vi "SERIAL_CapturePacket.vi"(11 "Stream":string) -> (0 "Packet Located":bool, 1 "Packet Length":i32, 2 "Packet":string, 3 "Stream":string)   [LabVIEW 2014, in "navX-MXP IMU.lvlib"]
uses:
  navX-MXP IMU.lvlib
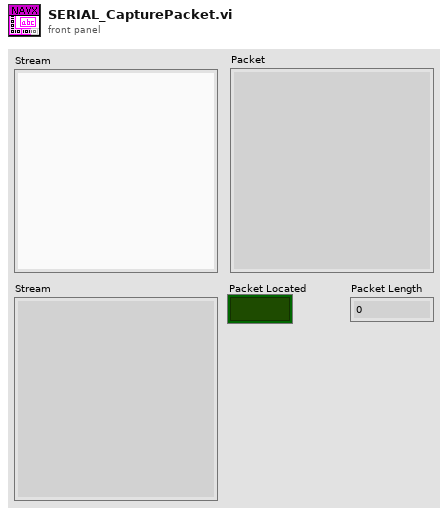
[diagram p1: front panel]
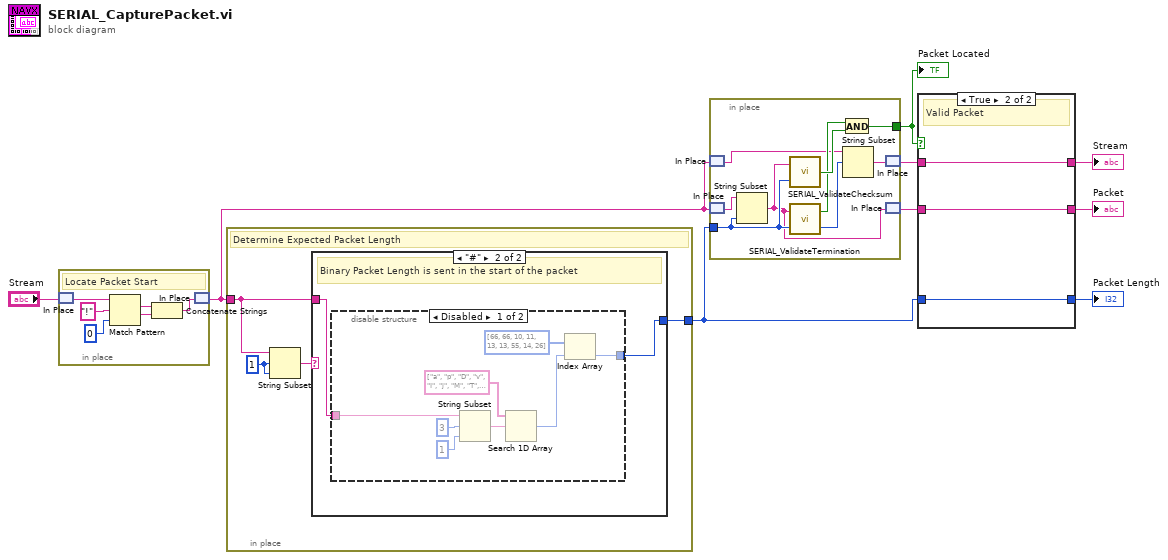
[diagram p0: block diagram]
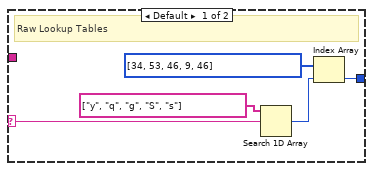
[diagram p2: hidden frame]
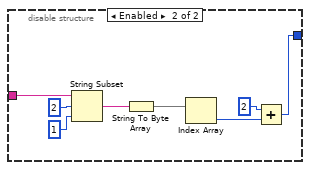
[diagram p3: hidden frame]
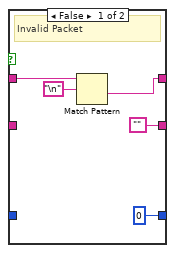
[diagram p4: hidden frame]
diagram:
  n1 = in-place {
    # "Locate Packet Start"
    n2 = in-place-match #1("Stream") -> (w11:string)
    n3 = Match Pattern(string=w11, regular expression="!" ("Packet Start Char"), offset (0)=0 ("offset past match")) -> (match substring=w14:string, after substring=w13:string)  [unwired: 2 out]
    n4 = Concatenate Strings(w14, w13) -> (w10:string)
    n5 = in-place-match #1(w10) -> (w3:string)
  }
  n6 = in-place {
    in-place-border: w3 -> [w18]
    in-place-border: [w17] -> w6
    w19 = 1 ("length (rest)")
    # "Determine Expected Packet Length"
    n7 = String Subset(string=w18, offset (0)=w19, length (rest)=w19) -> (substring=w16:string)
    n8 = case shown="\"#\"" w16 {
      selector: w16 -> [w20 _]
      tunnel: [w21 w26] -> w17
      tunnel: w18 -> [_ w25]
      frame Default {
        # "Raw Lookup Tables"
        n9 = Search 1D Array(1D array=string[] ["y", "q", "g", "S", "s"], element=w20) -> (index of element=w22:i32)  [unwired: 1 in]
        n10 = Index Array(array=i32[] [34, 53, 46, 9, 46], index=w22) -> (element=w21:i32)
      }
      frame "#" {
        # "Binary Packet Length is sent in the start of the packet"
        n11 = disable-structure shown="Disabled" {
          disable-tunnel: [w28 w35] -> w26
          disable-tunnel: w25 -> [w27 w36]
          frame Disabled {
            n12 = String Subset(string=w27, offset (0)=3, length (rest)=1 ("length (rest)")) -> (substring=w29:string)
            n13 = Search 1D Array(1D array=string[] ["a", "p", "D", "v", "I", "j", "M", "T", "i"], element=w29) -> (index of element=w34:i32)  [unwired: 1 in]
            n14 = Index Array(array=i32[] [66, 66, 10, 11, 13, 13, 55, 14, 26], index=w34) -> (element=w28:i32)
          }
          frame Enabled {
            n15 = String Subset(string=w36, offset (0)=2, length (rest)=1 ("length (rest)")) -> (substring=w39:string)
            n16 = String To Byte Array(string=w39) -> (unsigned byte array=w40:u8[])
            n17 = Index Array(array=w40) -> (element=w41:u8)  [unwired: 1 in]
            n18 = Add(x=u8 2 ("y"), y=w41) -> (x+y=w35:u8)
          }
        }
      }
    }
  }
  n19 = in-place {
    in-place-border: w6 -> [w50]
    in-place-border: [w47] -> w5
    n20 = in-place-match #2(w3) -> (w46:string)
    n21 = in-place-match #3(w3) -> (w45:string)
    n22 = String Subset(string=w45, length (rest)=w50) -> (substring=w43:string)  [unwired: 1 in]
    n23 = call "SERIAL_ValidateChecksum.vi"("Expected Packet Length"=w50, "Content"=w43) -> ("Valid?"=w49:bool)
    n24 = call "SERIAL_ValidateTermination.vi"("Expected Packet Length"=w50, "Content"=w43) -> ("Termination Offset"=w51:i32, "Valid?"=w48:bool)
    n25 = And(x=w48, y=w49) -> (x .and. y?=w47:bool)
    n26 = String Subset(string=w46, offset (0)=w51) -> (substring=w44:string)  [unwired: 1 in]
    n27 = in-place-match #2(w44) -> (w2:string)
    n28 = in-place-match #3(w43) -> (w1:string)
  }
  "Packet Located" <- w5
  n29 = case shown="True" w5 {
    tunnel: w2 -> [w56 w59]
    tunnel: [w55 w59] -> w8
    tunnel: w6 -> [_ w58]
    tunnel: [0 ("Packet Length") w58] -> w7
    tunnel: ["" w57] -> w9
    tunnel: w1 -> [_ w57]
    frame False {
      # "Invalid Packet"
      n30 = Match Pattern(string=w56, regular expression="\n") -> (after substring=w55:string)  [unwired: 1 in, 3 out]
    }
    frame True {
      # "Valid Packet"
    }
  }
  "Packet" <- w9
  "Stream" <- w8
  "Packet Length" <- w7
